vi "Dispose.vi"(8 "error in (no error)":errorcluster, 11 "EMKO":refnum<class "ESM-xx50.lvclass">) -> (0 "error out":errorcluster)   [LabVIEW 2022 SP3, in "EMKO.lvlib" / "ESM-xx50.lvclass"]
uses:
  ESM-xx50.lvclass
  ESM-xx50.lvclass/ESM-xx50.ctl
  <vilib>/Modbus/master/Modbus Master.lvclass
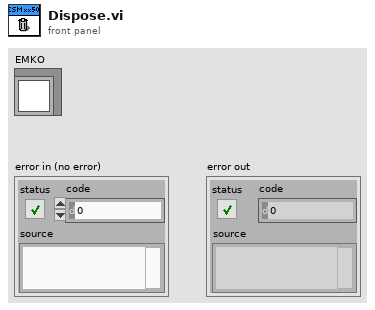
[diagram p1: front panel]
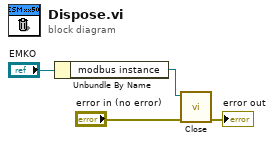
[diagram p0: block diagram]
diagram:
  n1 = Unbundle By Name("EMKO") -> ("modbus instance"=w3:refnum<class "Modbus Master.lvclass">)
  n2 = call-dynamic "Close.vi"("error in (no error)"="error in (no error)", "Modbus master in"=w3) -> ("error out"=→"error out":errorcluster)  [unwired: 9 in]
